vi "Read Manufacturer Data.vi"(7 "Unit ID (A)":string="A", 8 "error in":errorcluster, 11 "VISA Session In":refnum<visa-resource-name>="Alicat") -> (0 "error out":errorcluster, 1 "Manufacturer Info":string, 3 "VISA Session Out":refnum<visa-resource-name>)   [LabVIEW 2023]
doc: "Reads the manufacturing data from the specified Alicat device."
uses:
  <vilib>/Instr/_visa.llb/VISA Flush IO Buffer Mask.ctl
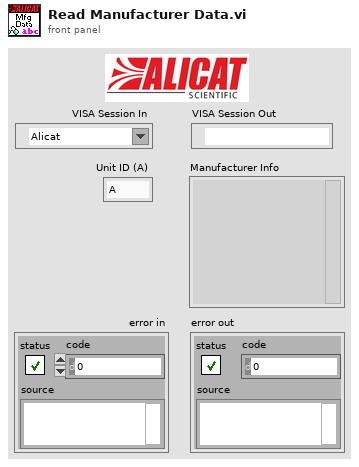
[diagram p1: front panel]
types:
  T1 = typedef "VISA Flush IO Buffer Mask.ctl" = u16
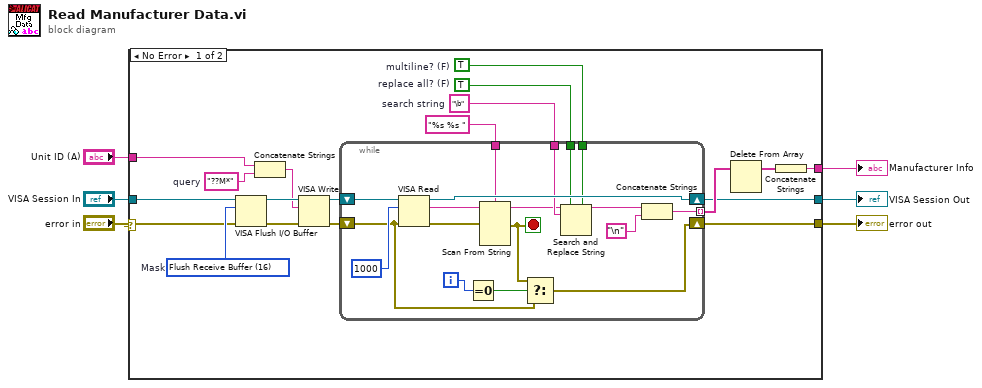
[diagram p0: block diagram]
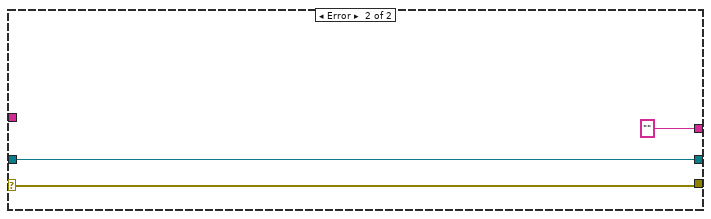
[diagram p2: hidden frame]
diagram:
  n1 = case shown="No Error" "error in" {
    selector: "error in" -> [w7 w44]
    tunnel: "VISA Session In" -> [w24 w45]
    tunnel: [w16 ""] -> w5
    tunnel: "Unit ID (A)" -> [w15 _]
    tunnel: [w9 w44] -> w3
    tunnel: [w8 w45] -> w2
    frame No Error {
      w14 = TRUE  # multiline? (F)
      w13 = TRUE  # replace all? (F)
      w12 = "\b"  # search string
      w19 = "??M*"  # query
      w22 = T1 16 items=["Flush Receive Buffer"=16, "Write Transmit Buffer to Device"=32, "Flush Receive Buffer (No I/O)"=64, "Flush Transmit Buffer"=128]  # Mask
      n2 = VISA Flush I/O Buffer(VISA resource name=w24, mask (16)=w22, error in (no error)=w7) -> (VISA resource name out=w23:refnum<visa-resource-name>, error out=w20:errorcluster)
      n3 = Concatenate Strings(w15, w19) -> (w18:string)
      n4 = VISA Write(VISA resource name=w23, write buffer=w18, error in (no error)=w20) -> (VISA resource name out=w21:refnum<visa-resource-name>, error out=w25:errorcluster)  [unwired: 1 out]
      n5 = while {
        tunnel: [w31] -> w10 mode=indexing
        shift-right: [w36] -> w9
        shift-left: w25 -> [w37]
        shift-right: [w41] -> w8
        shift-left: w21 -> [w43]
        tunnel: w14 -> [w35]
        tunnel: w13 -> [w34]
        tunnel: w12 -> [w33]
        tunnel: "%s %s " ("format string") -> [w32]
        i -> [w29]
        stop <- w30 stop-if-true
        n6 = VISA Read(VISA resource name=w43, byte count=u32 1000, error in (no error)=w37) -> (VISA resource name out=w41:refnum<visa-resource-name>, read buffer=w40:string, error out=w42:errorcluster)  [unwired: 1 out]
        n7 = Equal To 0?(x=w29) -> (x = 0?=w38:bool)
        n8 = Scan From String(format string=w32, input string=w40, error in=w42) -> (remaining string=w26:string, error out=w30:errorcluster)  [unwired: 5 in, 1 out]
        n9 = Select(t=w30, s=w38, f=w37) -> (s? t:f=w36:errorcluster)
        n10 = Search and Replace String(replace all?=w34, multiline?=w35, input string=w26, search string=w33) -> (result string=w27:string)  [unwired: 4 in, 3 out]
        n11 = Concatenate Strings(w27, "\n") -> (w31:string)
      }
      n12 = Delete From Array(array=w10) -> (array with subset deleted=w17:string[])  [unwired: 2 in, 1 out]
      n13 = Concatenate Strings(w17) -> (w16:string)
    }
    frame Error {
    }
  }
  "error out" <- w3
  "VISA Session Out" <- w2
  "Manufacturer Info" <- w5
